vi "Actuation.vi"() -> ()   [LabVIEW 2015]
uses:
  <vilib>/DAQmx/write.llb/DAQmx Write (Analog 1D Wfm NChan NSamp).vi
  <vilib>/DAQmx/create/channels.llb/DAQmx Create Channel (AO-Voltage-Basic).vi
  <vilib>/DAQmx/configure/timing.llb/DAQmx Timing (Sample Clock).vi
  <vilib>/DAQmx/miscellaneous.llb/DAQmx Fill In Error Info.vi
  <vilib>/measure/NI_MABase.lvlib
panel:
  in  "Start of Laser 2(2)":dbl format="%#_13g"
  in  "Pulse duration Laser 2 (2) (ms)":dbl=50.0 format="%0.2f"
  in  "Pulse duration Laser  1(2) (ms)  2":dbl
  in  "Start of Laser 1(2) 2":dbl format="%#_13g"
  in  "physical channels":tag
  in  "Pulse duration Laser  1 (ms)":dbl
  in  "Pulse duration Laser 2 (ms)":dbl=50.0 format="%0.2f"
  in  "Start of Laser 2":dbl format="%#_13g"
  in  "Start of Laser 1":dbl format="%#_13g"
  out "Waveform Graph":waveform(dbl)[](graph)
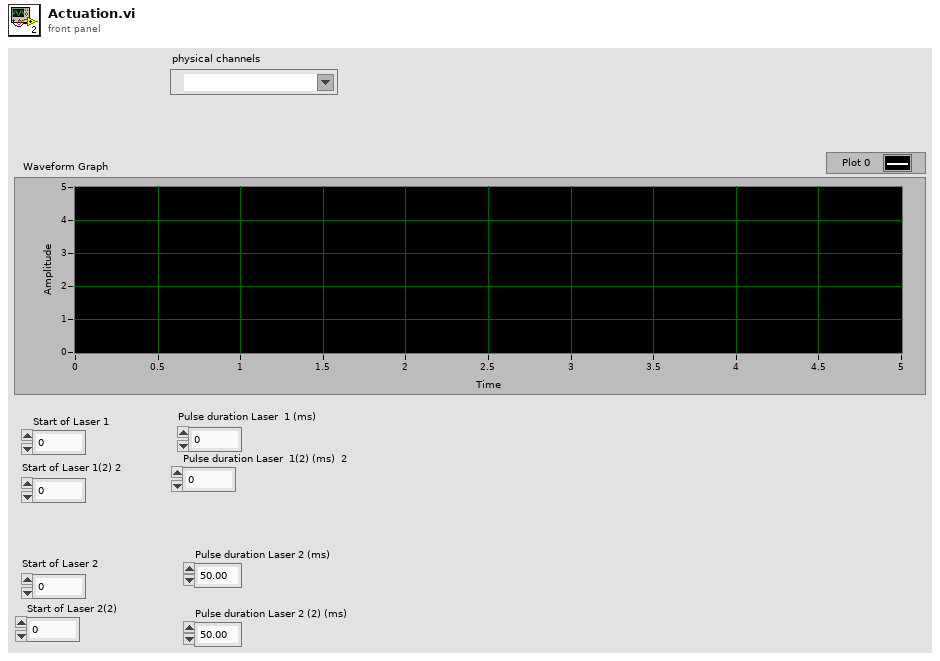
[diagram p1: front panel]
types:
  T1 = enum16{"Sine Wave", "Triangle Wave", "Square Wave", "Sawtooth Wave"}
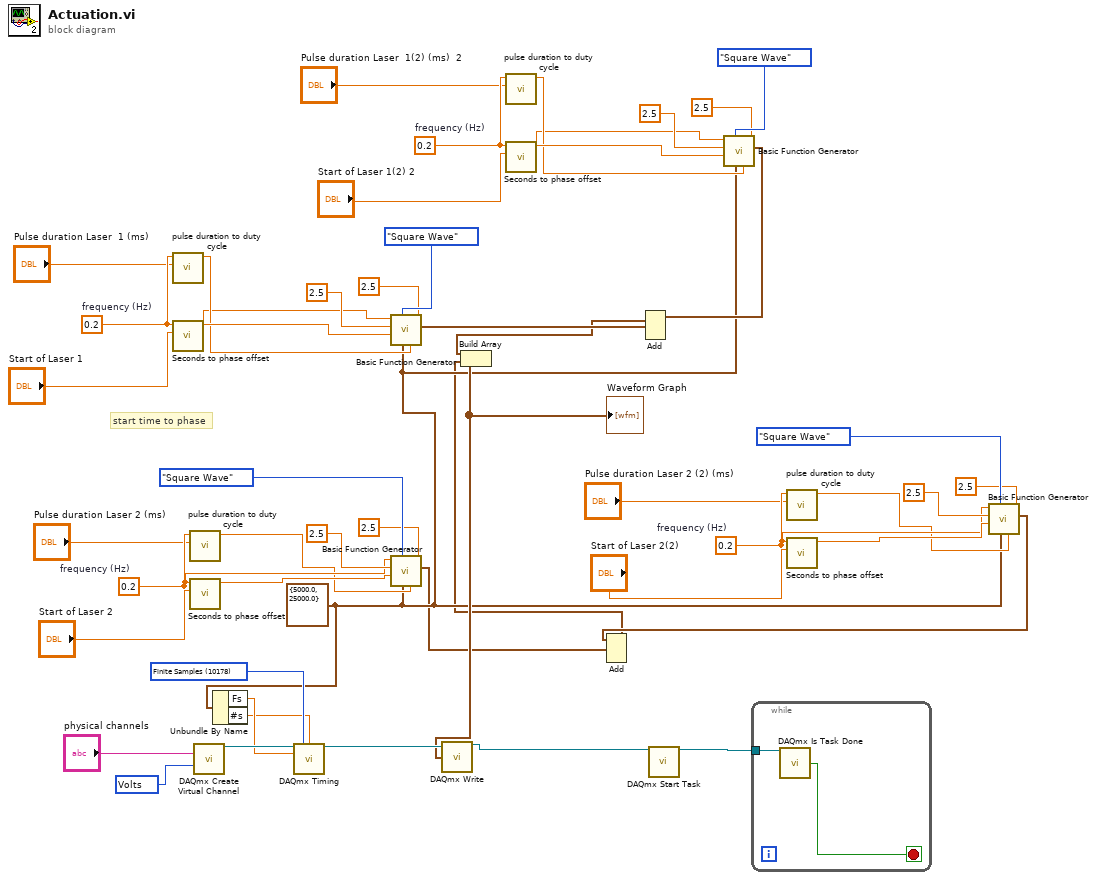
[diagram p0: block diagram]
diagram:
  w8 = 0.2  # frequency (Hz)
  w18 = 0.2  # frequency (Hz)
  w30 = 10178 items=["Finite Samples"=10178, "Continuous Samples"=10123, "Hardware Timed Single Point"=12522] ("sample mode")
  w33 = 10348 items=["Volts"=10348, "From Custom Scale"=10065] ("units")
  w4 = cluster{"Fs":dbl, "#s":dbl} {"Fs"=5000.0, "#s"=25000.0} ("sampling info")
  w39 = 0.2  # frequency (Hz)
  w35 = 0.2  # frequency (Hz)
  # "start time to phase"
  n1 = call "pulse duration to duty cycle.vi"("Pulse duration Laser  (ms)"="Pulse duration Laser  1 (ms)", "frequency"=w35) -> ("% duty cyle"=w36:dbl)  [unwired: 9 in]
  n2 = call "Seconds to phase offset.vi"("Start of Laser"="Start of Laser 1", "frequency"=w35) -> ("Phase"=w42:dbl)  [unwired: 9 in]
  n3 = call "pulse duration to duty cycle.vi"("Pulse duration Laser  (ms)"="Pulse duration Laser 2 (ms)", "frequency"=w39) -> ("% duty cyle"=w37:dbl)  [unwired: 9 in]
  n4 = call "Seconds to phase offset.vi"("Start of Laser"="Start of Laser 2", "frequency"=w39) -> ("Phase"=w41:dbl)  [unwired: 9 in]
  n5 = call-poly <vilib>:"DAQmx Create Virtual Channel.vi"("physical channels"="physical channels", "units"=w33) -> ("task out"=w31:refnum<k21>)  [unwired: 12 in, 1 out]
  n6 = Unbundle By Name(w4) -> ("Fs"=w29:dbl, "#s"=w28:dbl)
  n7 = call-poly <vilib>:"DAQmx Timing.vi"("task/channels in"=w31, "sample mode"=w30, "samples per channel"=w28, "rate"=w29) -> ("task out"=w26:refnum<k21>)  [unwired: 10 in, 1 out]
  n8 = call <vilib>:"Basic Function Generator.vi"("offset"=2.5, "square wave duty cycle (%)"=w36, "sampling info"=w4, "signal type"=T1."Square Wave", "phase"=w42, "amplitude"=2.5, "frequency"=w35) -> ("signal out"=w16:waveform(dbl))  [unwired: 2 in, 2 out]
  n9 = call <vilib>:"Basic Function Generator.vi"("offset"=2.5, "square wave duty cycle (%)"=w37, "sampling info"=w4, "signal type"=T1."Square Wave", "phase"=w41, "amplitude"=2.5, "frequency"=w39) -> ("signal out"=w3:waveform(dbl))  [unwired: 2 in, 2 out]
  n10 = call "pulse duration to duty cycle.vi"("Pulse duration Laser  (ms)"="Pulse duration Laser  1(2) (ms)  2", "frequency"=w18) -> ("% duty cyle"=w19:dbl)  [unwired: 9 in]
  n11 = call "Seconds to phase offset.vi"("Start of Laser"="Start of Laser 1(2) 2", "frequency"=w18) -> ("Phase"=w20:dbl)  [unwired: 9 in]
  n12 = call <vilib>:"Basic Function Generator.vi"("offset"=2.5, "square wave duty cycle (%)"=w19, "sampling info"=w4, "signal type"=T1."Square Wave", "phase"=w20, "amplitude"=2.5, "frequency"=w18) -> ("signal out"=w17:waveform(dbl))  [unwired: 2 in, 2 out]
  n13 = Add(1:w16, 2:w17) -> (0:w15:waveform(dbl))  [unwired: 1 in, 1 out]
  n14 = call "pulse duration to duty cycle.vi"("Pulse duration Laser  (ms)"="Pulse duration Laser 2 (2) (ms)", "frequency"=w8) -> ("% duty cyle"=w7:dbl)  [unwired: 9 in]
  n15 = call "Seconds to phase offset.vi"("Start of Laser"="Start of Laser 2(2)", "frequency"=w8) -> ("Phase"=w9:dbl)  [unwired: 9 in]
  n16 = call <vilib>:"Basic Function Generator.vi"("offset"=2.5, "square wave duty cycle (%)"=w7, "sampling info"=w4, "signal type"=T1."Square Wave", "phase"=w9, "amplitude"=2.5, "frequency"=w8) -> ("signal out"=w2:waveform(dbl))  [unwired: 2 in, 2 out]
  n17 = Add(1:w3, 2:w2) -> (0:w1:waveform(dbl))  [unwired: 1 in, 1 out]
  n18 = Build Array "Build Array"(w15, w1) -> (w25:waveform(dbl)[])
  "Waveform Graph" <- w25
  n19 = call-poly <vilib>:"DAQmx Write.vi"("task/channels in"=w26, "data"=w25) -> ("task out"=w24:refnum<k21>)  [unwired: 11 in, 2 out]
  n20 = call <vilib>:"DAQmx Start Task.vi"("task/channels in"=w24) -> ("task out"=w27:refnum<k21>)  [unwired: 13 in, 1 out]
  n21 = while {
    tunnel: w27 -> [w51]
    stop <- w50 stop-if-true
    n22 = call <vilib>:"DAQmx Is Task Done.vi"("task/channels in"=w51) -> ("task done?"=w50:bool)  [unwired: 12 in, 2 out]
  }
